vi "HomeAllAxes (SubVI).vi"(8 "error in (no error)":errorcluster) -> (0 "error out":errorcluster, 2 "Homed coordinates":T1, 3 "completed":bool)   [LabVIEW 2016]
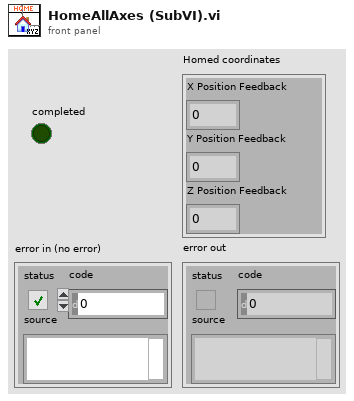
[diagram p1: front panel]
types:
  T1 = cluster{"X Position Feedback":dbl, "Y Position Feedback":dbl, "Z Position Feedback":dbl}
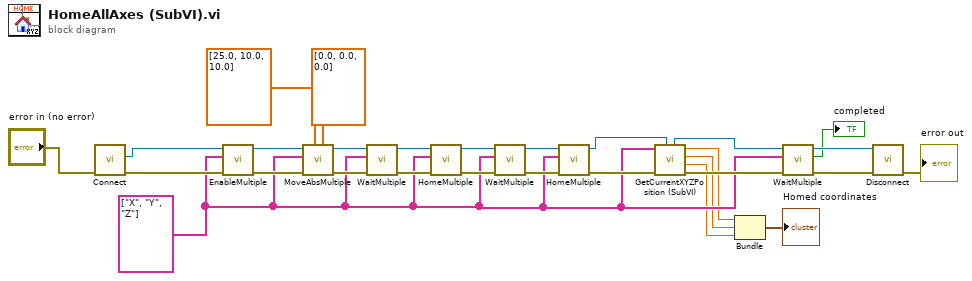
[diagram p0: block diagram]
diagram:
  w5 = string[] ["X", "Y", "Z"] ("axis names")
  n1 = call "Connect.vi"("error in (no error)"="error in (no error)") -> ("error out"=w26:errorcluster, "controller"=w27:refnum<k24>)  [unwired: 9 in]
  n2 = call "EnableMultiple.vi"("error in (no error)"=w26, "axis names"=w5, "controller in"=w27) -> ("error out"=w22:errorcluster, "controller out"=w23:refnum<k24>)  [unwired: 7 in]
  n3 = call "MoveAbsMultiple.vi"("positions"=dbl[] [0.0, 0.0, 0.0], "speeds"=dbl[] [25.0, 10.0, 10.0], "error in (no error)"=w22, "axis names"=w5, "controller in"=w23) -> ("error out"=w21:errorcluster, "controller out"=w20:refnum<k24>)  [unwired: 5 in]
  n4 = call "WaitMultiple.vi"("error in (no error)"=w21, "axis names"=w5, "controller in"=w20) -> ("error out"=w18:errorcluster, "controller out"=w19:refnum<k24>)  [unwired: 6 in, 1 out]
  n5 = call "HomeMultiple.vi"("error in (no error)"=w18, "axis names"=w5, "controller in"=w19) -> ("error out"=w16:errorcluster, "controller out"=w17:refnum<k24>)  [unwired: 7 in]
  n6 = call "WaitMultiple.vi"("error in (no error)"=w16, "axis names"=w5, "controller in"=w17) -> ("error out"=w14:errorcluster, "controller out"=w15:refnum<k24>)  [unwired: 6 in, 1 out]
  n7 = call "HomeMultiple.vi"("error in (no error)"=w14, "axis names"=w5, "controller in"=w15) -> ("error out"=w13:errorcluster, "controller out"=w12:refnum<k24>)  [unwired: 7 in]
  n8 = call "GetCurrentXYZPosition (SubVI).vi"(".NET Refnum in - Device"=w12, "error in (no error)"=w13, "Axes Names"=w5) -> ("error out"=w6:errorcluster, "Z Position Feedback"=w2:dbl, "Y Position Feedback"=w3:dbl, "X Position Feedback"=w4:dbl, ".NET Refnum out  - Device"=w7:refnum<k24>)  [unwired: 3 in]
  n9 = Bundle("X Position Feedback"=w4, "Y Position Feedback"=w3, "Z Position Feedback"=w2) -> (→"Homed coordinates":T1)  [unwired: 1 in]
  n10 = call "WaitMultiple.vi"("error in (no error)"=w6, "axis names"=w5, "controller in"=w7) -> ("error out"=w8:errorcluster, "completed"=→"completed":bool, "controller out"=w10:refnum<k24>)  [unwired: 6 in]
  n11 = call "Disconnect.vi"("error in (no error)"=w8, "controller"=w10) -> ("error out"=→"error out":errorcluster)  [unwired: 9 in]
